vi "svl_Max-Min Resampled Level (N Ch).vi"(8 "error in (no error)":errorcluster, 9 "processing state":T1(ring), 11 "even angle signals":T2(array[cluster]) {"even angle signal" format="%.2f"; "dr" format="%.2f"; "r0" format="%.2f"}) -> (0 "error out":errorcluster, 1 "max-min level(s)":dbl[](array[numeric]) format="%.2f", 2 "min level(s)":dbl[](array[numeric]) format="%.2f", 3 "max level(s)":dbl[](array[numeric]) format="%.2f")   [LabVIEW 2017]
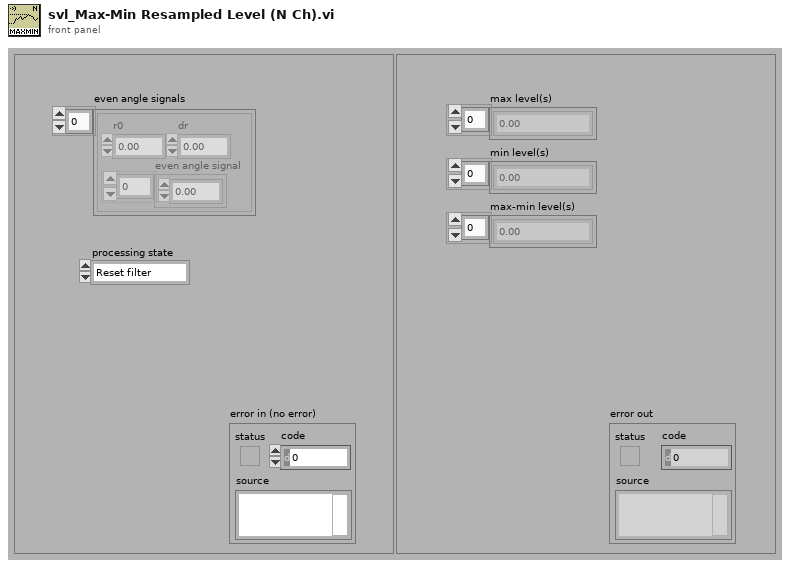
[diagram p1: front panel]
types:
  T1 = enum16{"Reset filter", "Restart averaging", "Continue processing"}
  T2 = cluster{"r0":dbl, "dr":dbl, "even angle signal":dbl[]}[]
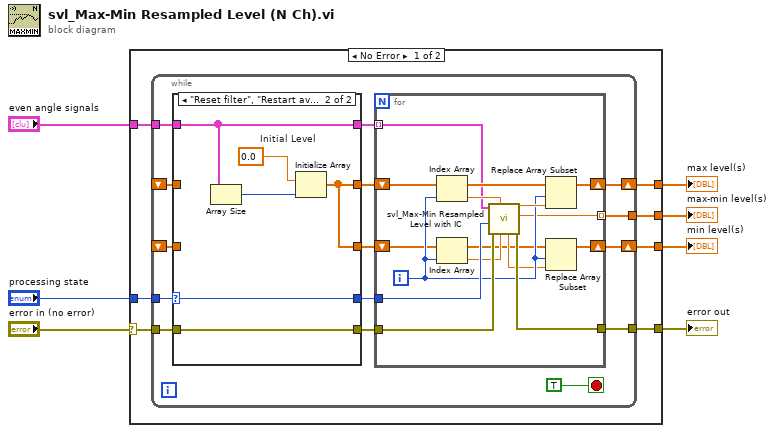
[diagram p0: block diagram]
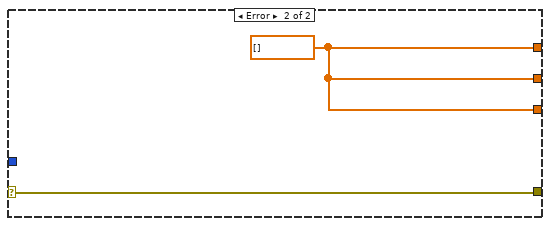
[diagram p3: hidden frame]
diagram:
  n1 = case shown="No Error" "error in (no error)" {
    selector: "error in (no error)" -> [w12 w56]
    tunnel: "processing state" -> [w14 _]
    tunnel: "even angle signals" -> [w13 _]
    tunnel: [w10 w55] -> w5
    tunnel: [w11 w56] -> w3
    tunnel: [w9 w55] -> w2
    tunnel: [w8 w55] -> w1
    frame No Error {
      n2 = while {
        tunnel: [w21] -> w11
        tunnel: w12 -> [w20]
        shift-left: _ -> [w25]
        shift-right: [w28] -> w10
        tunnel: w13 -> [w23]
        tunnel: w14 -> [w27]
        shift-right: [w18] -> w9
        shift-left: _ -> [w17]
        tunnel: [w15] -> w8
        stop <- TRUE stop-if-true
        n3 = case shown="\"Reset filter\", \"Restart averaging\"" w27 {
          selector: w27 -> [w34 w40]
          tunnel: [w34 w40] -> w26
          tunnel: w25 -> [w33 _]
          tunnel: [w33 w36] -> w24
          tunnel: w23 -> [w32 w39]
          tunnel: [w32 w39] -> w22
          tunnel: w20 -> [w31 w38]
          tunnel: [w31 w38] -> w19
          tunnel: w17 -> [w30 _]
          tunnel: [w30 w36] -> w16
          frame "Continue processing", Default {
          }
          frame "Reset filter", "Restart averaging" {
            w37 = 0.0  # Initial Level
            n4 = Array Size(array=w39) -> (size(s)=w35:i32)
            n5 = Initialize Array(w37, w35) -> (w36:dbl[])
          }
        }
        n6 = for {
          tunnel: w22 -> [w41] mode=indexing
          shift-right: [w54] -> w28
          shift-left: w24 -> [w53]
          tunnel: w26 -> [w50]
          tunnel: w19 -> [w52]
          tunnel: [w51] -> w21
          shift-right: [w46] -> w18
          shift-left: w16 -> [w42]
          tunnel: [w43] -> w15 mode=indexing
          i -> [w47]
          n7 = Index Array(array=w53, index=w47) -> (element=w48:dbl)
          n8 = Index Array(array=w42, index=w47) -> (element=w44:dbl)
          n9 = call <vilib>:"svl_Max-Min Resampled Level with IC.vi"("initial min level"=w44, "initial max level"=w48, "error in (no error)"=w52, "processing state"=w50, "even angle signal"=w41) -> ("error out"=w51:errorcluster, "max-min level"=w43:dbl, "final min level"=w45:dbl, "final max level"=w49:dbl)  [unwired: 3 in]
          n10 = Replace Array Subset(array=w53, new element=w49, index=w47) -> (w54:dbl[])
          n11 = Replace Array Subset(array=w42, new element=w45, index=w47) -> (w46:dbl[])
        }
      }
    }
    frame Error {
      w55 = dbl[] []
    }
  }
  "max level(s)" <- w5
  "error out" <- w3
  "min level(s)" <- w2
  "max-min level(s)" <- w1
